vi "Main_Program_with_RFSA.vi"() -> ()   [LabVIEW 2014]
uses:
  15_DataManagement/Device_Resources.ctl
panel:
  in  "Device Resources":T1={"RFSG Resource in"="VST", "RFSA Resource in"="VST", "RFmx Resource in"="VST"}
  # "[ Gyuwon Main ]"
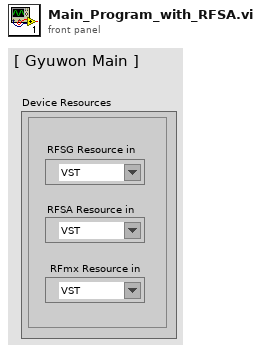
[diagram p1: front panel]
types:
  T1 = typedef "Device_Resources.ctl" = cluster{"RFSG Resource in":refnum<k15>, "RFSA Resource in":refnum<k15>, "RFmx Resource in":refnum<k15>}
  T2 = typedef "Message_Queues.ctl" = cluster{"RFSG_QTx":refnum<queue>, "RFSG_QRx":refnum<queue>, "RFSA_QTx":refnum<queue>, "RFSA_QRx":refnum<queue>, "SysLog":refnum<queue>, "RFSA_Data":refnum<queue>, "RFmx_QTx":refnum<queue>, "RFmx_QRx":refnum<queue>, "RFmx_Data":refnum<queue>}
  T3 = enum32{"Invalid", "Standard", "Closed", "Hidden", "Minimized", "Maximized"}
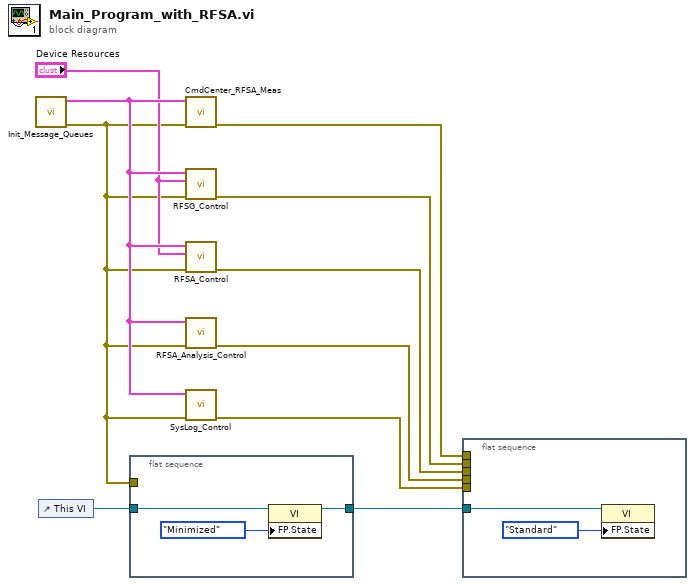
[diagram p0: block diagram]
diagram:
  n1 = call "Init_Message_Queues.vi"() -> ("error out"=w6:errorcluster, "Queue_Out"=w10:T2)  [unwired: 10 in]
  n2 = control-ref of="This VI"() -> (w8:refnum<vi>)
  n3 = flat-sequence {
    tunnel: w8 -> [w13]
    tunnel: w6 -> [_]
    tunnel: [w11] -> w7
    frame #0 {
      n4 = property class="VI"(reference=w13, "FP.State"=T3."Minimized" ("Front Panel Window:State")) -> (reference out=w11:refnum<vi>)  [unwired: 1 in, 1 out]
    }
  }
  n5 = call "CmdCenter_RFSA_Meas.vi"("error in (no error)"=w6, "Message_Queues"=w10) -> ("error out"=w1:errorcluster)  [unwired: 9 in]
  n6 = call "RFSG_Control.vi"("error in (no error)"=w6, "Device Resources"="Device Resources", "Message_Queues"=w10) -> ("error out"=w2:errorcluster)  [unwired: 8 in]
  n7 = call "RFSA_Control.vi"("error in (no error)"=w6, "Device Resources"="Device Resources", "Message_Queues"=w10) -> ("error out"=w3:errorcluster)  [unwired: 8 in]
  n8 = call "RFSA_Analysis_Control.vi"("error in (no error)"=w6, "Message_Queues"=w10) -> ("error out"=w4:errorcluster)  [unwired: 9 in]
  n9 = call "SysLog_Control.vi"("error in (no error)"=w6, "Message_Queues"=w10) -> ("error out"=w5:errorcluster)  [unwired: 9 in]
  n10 = flat-sequence {
    tunnel: w7 -> [w16]
    tunnel: w3 -> [_]
    tunnel: w4 -> [_]
    tunnel: w5 -> [_]
    tunnel: w2 -> [_]
    tunnel: [w14] -> _
    tunnel: w1 -> [w14]
    frame #0 {
      n11 = property class="VI"(reference=w16, "FP.State"=T3."Standard" ("Front Panel Window:State")) -> ()  [unwired: 1 in, 2 out]
    }
  }
